vi "RVC Euler Transformation.vi"() -> ()   [LabVIEW 2013]
uses:
  <vilib>/Analysis/coordinate.llb/Euler Rotation Order.ctl
  <vilib>/robotics/Kinematics/NI_Kinematics.lvlib
  <vilib>/Analysis/NI_AALPro.lvlib
panel:
  in  "type of transformation":u16(ring) items=["active (alibi)", "passive (alias)"]
  in  "Stop":bool
  in  "rotation order":T1=11 items=["X-Y-Z", "X-Z-Y", "Y-X-Z", "Y-Z-X", "Z-X-Y", "Z-Y-X", "X-Y-X", "X-Z-X", "Y-X-Y", "Y-Z-Y", "Z-X-Z", "Z-Y-Z"]
  in  "type of rotations":u16(ring) items=["Extrinsic", "Intrinsic"]
  out "gamma (euler angles)":cluster{"phi":dbl, "theta":dbl, "psi":dbl}={"phi"=0.10000000000000009, "theta"=0.2, "psi"=0.2999999999999998}
  out "transformation matrix":picture
  in  "Position":dbl[](array[numeric])=[1.0, 1.0, 1.0]
  in  "angles":cluster{"phi":dbl, "theta":dbl, "psi":dbl}={"phi"=0.1, "theta"=0.2, "psi"=0.3} {"phi" scale=-3.14..3.14; "theta" scale=-1.54..1.54; "psi" scale=-3.14..3.14}
  out "3D Picture":refnum<vi>(3d-picture)
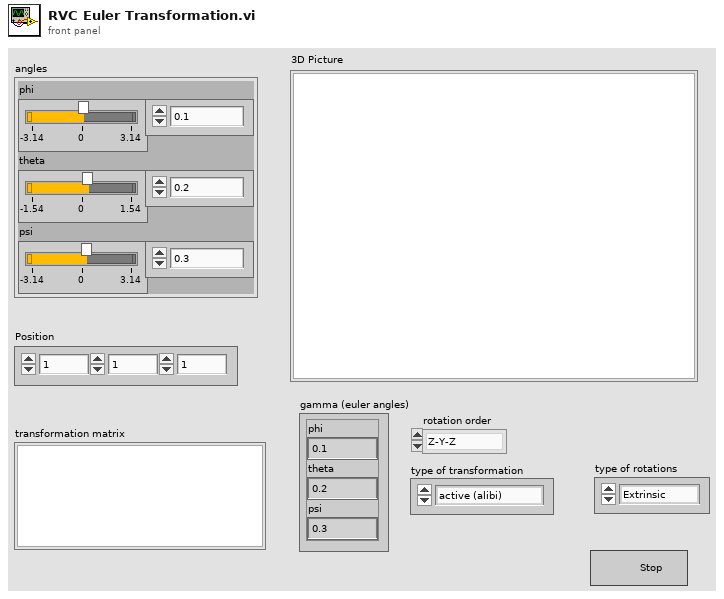
[diagram p1: front panel]
types:
  T1 = typedef "NI_AALPro.lvlib/Euler Rotation Order.ctl" = u16
  T2 = typedef "NI_Matrix.lvlib/RealMatrix.ctl" = dbl[][]
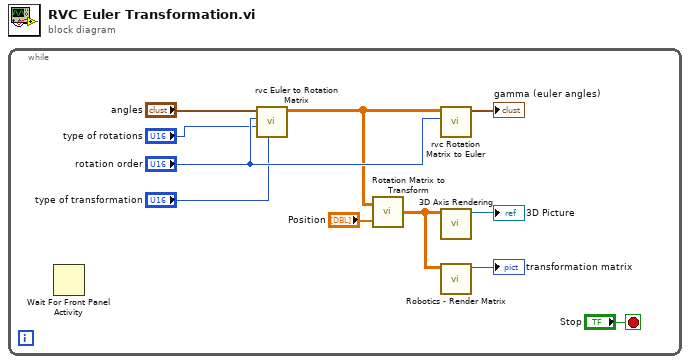
[diagram p0: block diagram]
diagram:
  n1 = while {
    stop <- "Stop" stop-if-true
    n2 = Wait For Front Panel Activity() -> ()  [unwired: 3 in, 1 out]
    n3 = call "rvc Euler to Rotation Matrix.vi"("type of transformation"="type of transformation", "type of rotations"="type of rotations", "rotation order"="rotation order", "euler angles"="angles") -> ("rotation matrix"=w5:T2)  [unwired: 6 in, 1 out]
    n4 = call <vilib>:"Rotation Matrix to Transform.vi"("translation vector"="Position", "rotation matrix"=w5) -> ("transform"=w1:T2)
    n5 = call "rvc Rotation Matrix to Euler.vi"("rotation order"="rotation order", "rotation matrix"=w5) -> ("euler angles"=→"gamma (euler angles)":cluster{"phi":dbl, "theta":dbl, "psi":dbl})  [unwired: 8 in, 1 out]
    n6 = call "3D Axis Rendering.vi"("rotation matrix"=w1) -> ("SceneNode out"=→"3D Picture":refnum<vi>)  [unwired: 9 in, 1 out]
    n7 = call "Robotics - Render Matrix.vi"("A"=w1) -> ("picture out"=→"transformation matrix":picture)  [unwired: 10 in]
  }
